vi "Cover Engine.vi"(0 "Current Minefield":picture, 5 "Minefield Base Picture":picture, 7 "Cover Operation":T1, 9 "Operation Index (row, column)":cluster{"x":i16, "y":i16}, 11 "Error In":errorcluster) -> (4 "Minefield Picture Out":picture, 15 "Error Out":errorcluster)   [LabVIEW 2011]
doc: "Returns a new minefield picture as the result of a command given as an enumerated type that acts on a specific index. Commands include cover, uncover, flag, and unflag. The base minefield picture is needed for uncover operations."
uses:
  Cover Operation Typdef.ctl
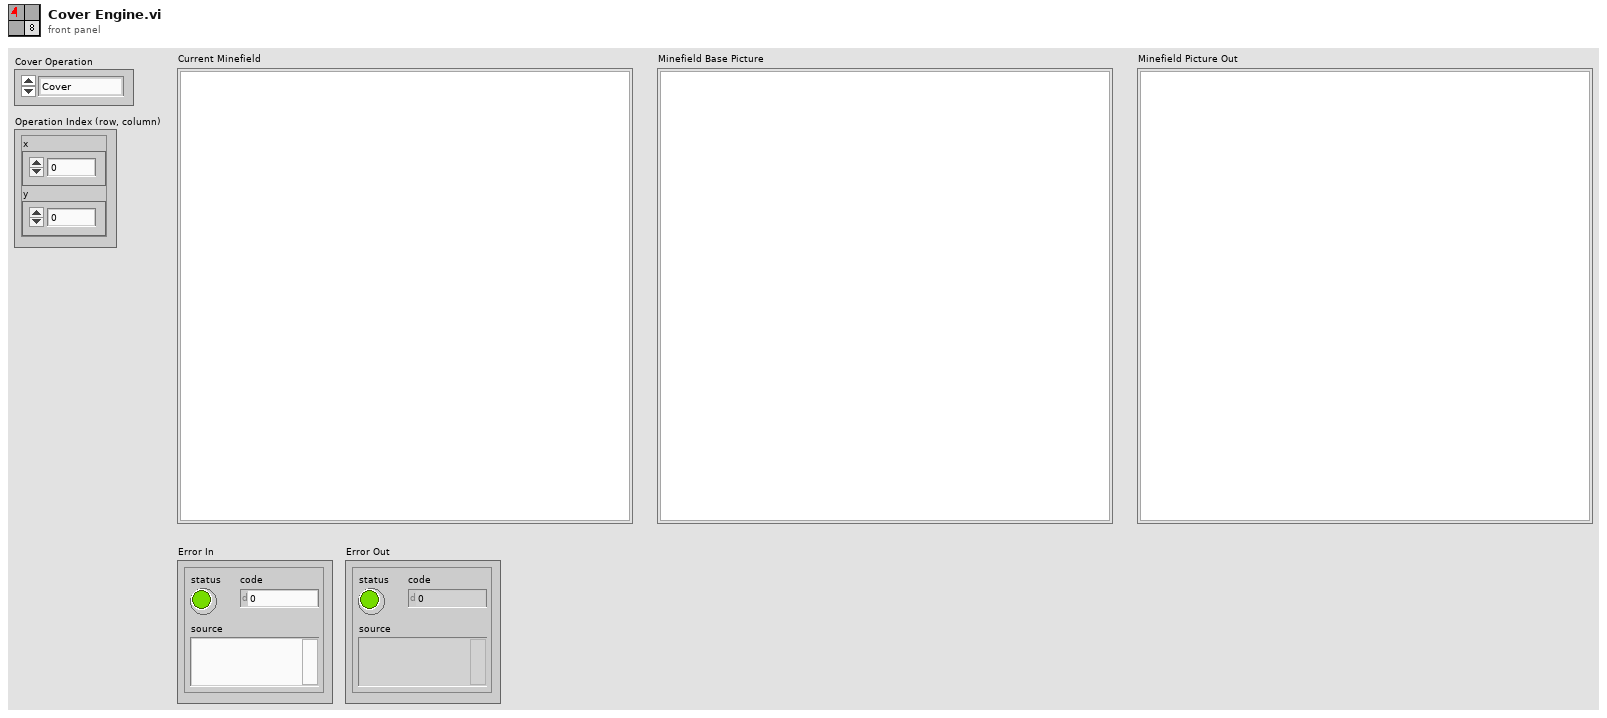
[diagram p1: front panel]
types:
  T1 = typedef "Cover Operation Typdef.ctl" = enum16{"Cover", "Uncover", "Flag", "Unflag"}
  T2 = typedef "imagedata.ctl" = cluster{"image type":i32, "image depth":i32, "image":u8[], "mask":u8[], "colors":u32[], "Rectangle":cluster{"left":i16, "top":i16, "right":i16, "bottom":i16}}
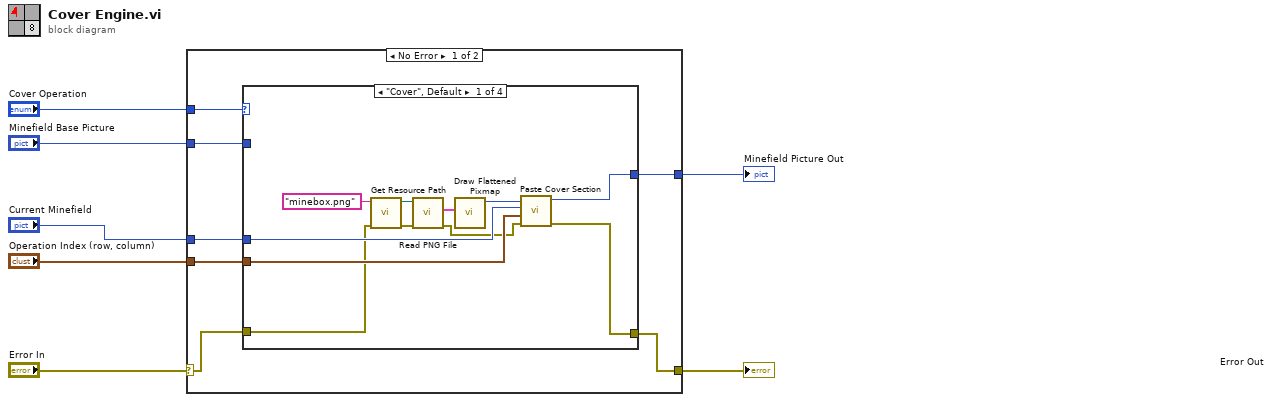
[diagram p0: block diagram]
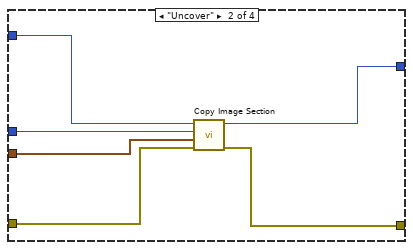
[diagram p2: hidden frame]
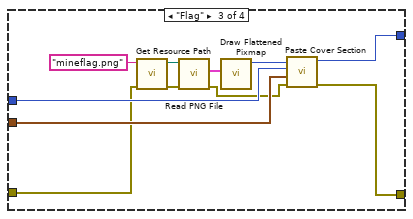
[diagram p3: hidden frame]
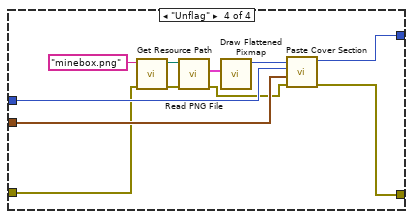
[diagram p4: hidden frame]
diagram:
  n1 = case shown="No Error" "Error In" {
    selector: "Error In" -> [w8 w54]
    tunnel: "Current Minefield" -> [w14 w55]
    tunnel: "Minefield Base Picture" -> [w13 _]
    tunnel: [w12 w55] -> w5
    tunnel: [w11 w54] -> w4
    tunnel: "Operation Index (row, column)" -> [w10 _]
    tunnel: "Cover Operation" -> [w9 _]
    frame No Error {
      n2 = case shown="\"Cover\", Default" w9 {
        tunnel: w14 -> [w21 w31 w38 w49]
        tunnel: w13 -> [_ w30 _ _]
        tunnel: [w17 w29 w34 w45] -> w12
        tunnel: [w18 w28 w35 w46] -> w11
        tunnel: w10 -> [w20 w27 w37 w48]
        tunnel: w8 -> [w16 w26 w32 w44]
        frame "Cover", Default {
          n3 = call "Get Resource Path.vi"("Error In"=w16, "Resource Filename"="minebox.png" ("resource filename")) -> ("Error Out"=w15:errorcluster, "Resource Path"=w24:path)  [unwired: 8 in]
          n4 = call <vilib>:"Read PNG File.vi"("error in (no error)"=w15, "path to PNG file"=w24) -> ("error out"=w19:errorcluster, "image data"=w25:T2)  [unwired: 7 in, 1 out]
          n5 = call <vilib>:"Draw Flattened Pixmap.vi"("image data"=w25) -> ("new picture"=w22:picture)  [unwired: 8 in]
          n6 = call "Paste Cover Section.vi"("Error In"=w19, "Mine Index (row, column)"=w20, "Pasteboard Picture"=w21, "Cover Picture"=w22) -> ("Error Out"=w18:errorcluster, "Output Picture"=w17:picture)  [unwired: 6 in]
        }
        frame "Uncover" {
          n7 = call "Copy Image Section.vi"("Error In"=w26, "Index to Copy (row, column)"=w27, "Pasteboard Picture"=w31, "Copy Picture"=w30) -> ("Error Out"=w28:errorcluster, "Output Picture"=w29:picture)  [unwired: 6 in]
        }
        frame "Flag" {
          n8 = call "Get Resource Path.vi"("Error In"=w32, "Resource Filename"="mineflag.png" ("resource filename")) -> ("Error Out"=w33:errorcluster, "Resource Path"=w41:path)  [unwired: 8 in]
          n9 = call <vilib>:"Read PNG File.vi"("error in (no error)"=w33, "path to PNG file"=w41) -> ("error out"=w36:errorcluster, "image data"=w42:T2)  [unwired: 7 in, 1 out]
          n10 = call <vilib>:"Draw Flattened Pixmap.vi"("image data"=w42) -> ("new picture"=w39:picture)  [unwired: 8 in]
          n11 = call "Paste Cover Section.vi"("Error In"=w36, "Mine Index (row, column)"=w37, "Pasteboard Picture"=w38, "Cover Picture"=w39) -> ("Error Out"=w35:errorcluster, "Output Picture"=w34:picture)  [unwired: 6 in]
        }
        frame "Unflag" {
          n12 = call "Get Resource Path.vi"("Error In"=w44, "Resource Filename"="minebox.png" ("resource filename")) -> ("Error Out"=w43:errorcluster, "Resource Path"=w52:path)  [unwired: 8 in]
          n13 = call <vilib>:"Read PNG File.vi"("error in (no error)"=w43, "path to PNG file"=w52) -> ("error out"=w47:errorcluster, "image data"=w53:T2)  [unwired: 7 in, 1 out]
          n14 = call <vilib>:"Draw Flattened Pixmap.vi"("image data"=w53) -> ("new picture"=w50:picture)  [unwired: 8 in]
          n15 = call "Paste Cover Section.vi"("Error In"=w47, "Mine Index (row, column)"=w48, "Pasteboard Picture"=w49, "Cover Picture"=w50) -> ("Error Out"=w46:errorcluster, "Output Picture"=w45:picture)  [unwired: 6 in]
        }
      }
    }
    frame Error {
    }
  }
  "Error Out" <- w4
  "Minefield Picture Out" <- w5
